vi "writeToXML.vi"(8 "error in (no error)":errorcluster, 10 "ClassLabel":string, 11 "CollimationOffsetCommands in":refnum<class "CollimationOffsetCommands.lvclass">) -> (0 "error out":errorcluster, 2 "XML out":string, 3 "CollimationOffsetCommands out":refnum<class "CollimationOffsetCommands.lvclass">)   [LabVIEW 2022 SP3, in "TCSDataDefinitions.lvlib" / "TCSCommand.lvlib" / "OffsetCommands.lvlib" / "CollimationOffsetCommands.lvclass"]
uses:
  CollimationOffsetCommands.lvclass
  OffsetCommands/OffsetCommands.lvclass
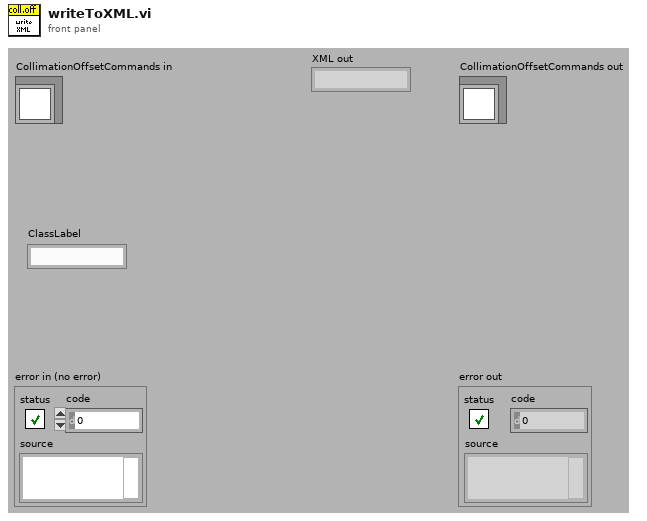
[diagram p1: front panel]
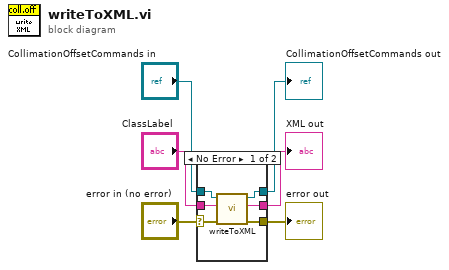
[diagram p0: block diagram]
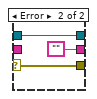
[diagram p2: hidden frame]
diagram:
  n1 = case shown="No Error" "error in (no error)" {
    selector: "error in (no error)" -> [w9 w15]
    tunnel: [w8 w15] -> w5
    tunnel: [w11 w14] -> w3
    tunnel: "CollimationOffsetCommands in" -> [w12 w14]
    tunnel: "ClassLabel" -> [w10 _]
    tunnel: [w7 ""] -> w1
    frame No Error {
      n2 = call-parent "writeToXML.vi"("error in (no error)"=w9, "ClassLabel"=w10, "OffsetCommands in"=w12) -> ("error out"=w8:errorcluster, "XML out"=w7:string, "OffsetCommands out"=w11:refnum<class "CollimationOffsetCommands.lvclass">)  [unwired: 6 in]
    }
    frame Error {
    }
  }
  "error out" <- w5
  "CollimationOffsetCommands out" <- w3
  "XML out" <- w1
